vi "TeOp.vi"   [LabVIEW 2017]
doc: "This VI is called for each TeleOp packet received from the DS where the robot is not disabled. It is often used to read from the joysticks and update I/O or to update setpoints for timed control loops. It should complete and return within 20 milliseconds or it may miss DS packets."
uses:
  TypeDef/ENUM_Joystick_Buttons.ctl
  TypeDef/ENUM_Joystick_Axes.ctl
  TypeDef/CLUSTER_CMD_WC_Drive.ctl
  TypeDef/ENUM_WC_Drive_DriveMode.ctl
  TypeDef/CLUSTER_Drive_ACT Loop_VBus Data.ctl
  TypeDef/CLUSTER_X and Y.ctl
  TypeDef/CLUSTER_Drive_ACT Loop_Profile Data.ctl
  Systems/Joystick/Global_Joystick Write_Data.vi
  Globals/Global_CMD_Gear.vi
  Globals/Global_CMD_Drive.vi
  Systems/Joystick/Joystick.lvlib
types:
  T1 = typedef "ENUM_Joystick_Buttons.ctl" = enum16{"Green A", "Red B", "Blue X", "Yellow Y", "Left Bumper", "Right Bumper", "Back", "Start", "Left Joystick", "Right Joystick"}
  T2 = typedef "CLUSTER_CMD_WC_Drive.ctl" = cluster{"Drive_Mode":T3, "VBus":T4, "Profile":T6}
  T3 = typedef "ENUM_WC_Drive_DriveMode.ctl" = enum16{"Motion Profile", "VBus", "Stop"}
  T4 = typedef "CLUSTER_Drive_ACT Loop_VBus Data.ctl" = cluster{"Drive":T5, "Turbo":bool}
  T5 = typedef "CLUSTER_X and Y.ctl" = cluster{"Steer":dbl, "Throtle":dbl}
  T6 = typedef "CLUSTER_Drive_ACT Loop_Profile Data.ctl" = cluster{"Start":bool}
  T7 = typedef "ENUM_Joystick_Axes.ctl" = enum16{"Left X", "Left Y", "Left Trigger", "Right Trigger", "Right X", "Right Y"}
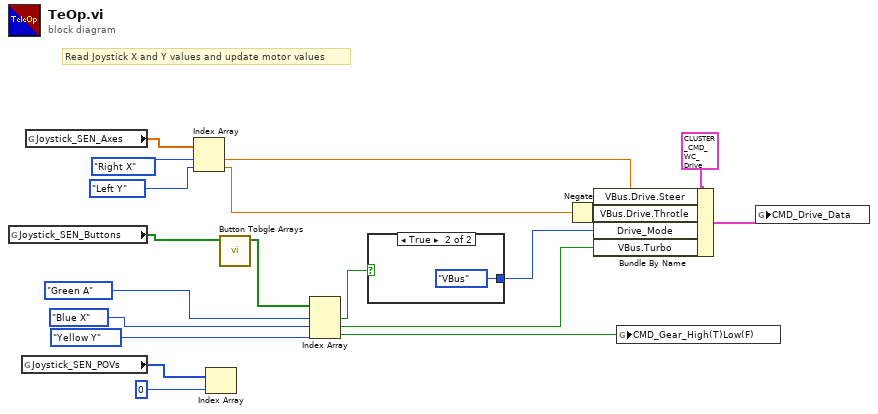
[diagram p0: block diagram]
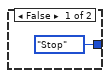
[diagram p2: hidden frame]
diagram:
  # "Read Joystick X and Y values and update motor values"
  n1 = global read "Global_Joystick Write_Data.vi" "Joystick_SEN_Buttons"() -> (w8:bool[])
  n2 = global read "Global_Joystick Write_Data.vi" "Joystick_SEN_POVs"() -> (w18:i16[])
  n3 = global read "Global_Joystick Write_Data.vi" "Joystick_SEN_Axes"() -> (w19:dbl[])
  n4 = Index Array(array=w19, index #1=ENUM_Joystick_Axes."Right X" ("Joystick_Axes"), index #2=ENUM_Joystick_Axes."Left Y" ("Joystick_Axes")) -> (element #1=w3:dbl, element #2=w1:dbl)
  n5 = Index Array(array=w18, index=0) -> ()  [unwired: 1 out]
  n6 = call "Button Tobgle Arrays.vi"("Joystick_SEN_Buttons"=w8) -> ("Toggle Outputs Out"=w11:bool[])  [unwired: 8 in, 2 out]
  n7 = Index Array(array=w11, index #1=ENUM_Joystick_Buttons."Green A" ("Joystick_Buttons"), index #2=ENUM_Joystick_Buttons."Blue X" ("Joystick_Buttons"), index #3=ENUM_Joystick_Buttons."Yellow Y" ("Joystick_Buttons")) -> (element #1=w10:bool, element #2=w6:bool, element #3=w4:bool)
  n8 = case shown="True" w10 {
    tunnel: [ENUM_WC_Drive_DriveMode."Stop" ("CMD_Drive_Mode") ENUM_WC_Drive_DriveMode."VBus" ("CMD_Drive_Mode")] -> w9
    frame False {
    }
    frame True {
    }
  }
  n9 = Negate(x=w1) -> (-x=w2:dbl)
  n10 = Bundle By Name(cluster=T2 {"Drive_Mode"=enum."Motion Profile", "VBus"={"Drive"={"Steer"=0.0, "Throtle"=0.0}, "Turbo"=FALSE}, "Profile"={"Start"=FALSE}} ("CMD_DriveCluster"), "VBus.Drive.Steer"=w3, "VBus.Drive.Throtle"=w2, "Drive_Mode"=w9, "VBus.Turbo"=w6) -> (w14:T2)
  n11 = global write "Global_CMD_Gear.vi" "CMD_Gear_High(T)Low(F)"(w4) -> ()
  n12 = global write "Global_CMD_Drive.vi" "CMD_Drive_Data"(w14) -> ()
